vi "exnFormulaBlock Express Formula Template.vi"(0 "X1":waveform(dbl)[](array[waveform]), 1 "X2":waveform(dbl)[](array[waveform]), 2 "X3":waveform(dbl)[](array[waveform]), 3 "X4":waveform(dbl)[](array[waveform]), 5 "X5":waveform(dbl)[](array[waveform]), 7 "X6":waveform(dbl)[](array[waveform]), 9 "X7":waveform(dbl)[](array[waveform]), 11 "error in (no error)":errorcluster, 12 "X8":waveform(dbl)[](array[waveform])) -> (8 "Result":waveform(dbl)[](array[waveform]), 15 "error out":errorcluster)   [LabVIEW 2020]
panel:
  in  "Name Modifier":string="Formula Result"
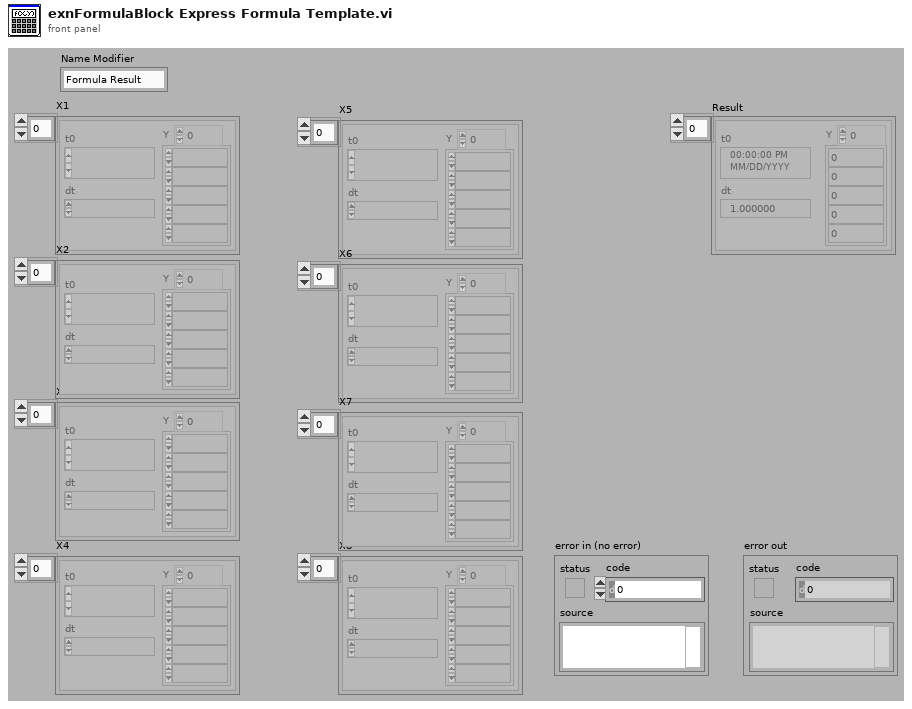
[diagram p1: front panel]
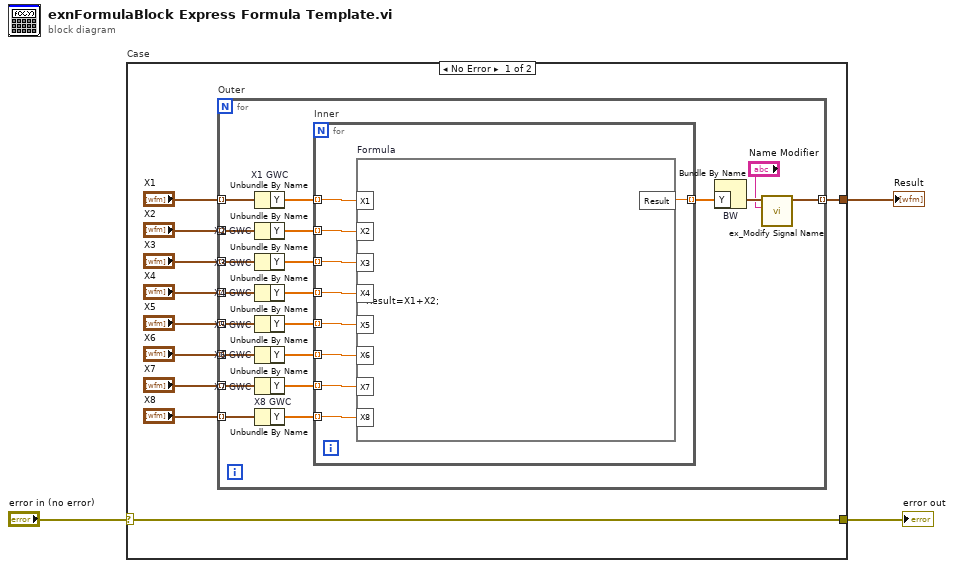
[diagram p0: block diagram]
diagram:
  n1 = case "Case" shown="No Error" "error in (no error)" {
    selector: "error in (no error)" -> [w4 w43]
    tunnel: [w5 _] -> w3
    tunnel: [w4 w43] -> w1
    frame No Error {
      n2 = for "Outer" {
        tunnel: "X1" -> [w33] mode=indexing
        tunnel: "X2" -> [w31] mode=indexing
        tunnel: "X3" -> [w23] mode=indexing
        tunnel: "X4" -> [w22] mode=indexing
        tunnel: "X5" -> [w21] mode=indexing
        tunnel: "X6" -> [w20] mode=indexing
        tunnel: "X7" -> [w19] mode=indexing
        tunnel: "X8" -> [w18] mode=indexing
        tunnel: [w15] -> w5 mode=indexing
        n3 = Unbundle By Name "X1 GWC"(w33) -> ("Y"=w32:dbl[])
        n4 = Unbundle By Name "X2 GWC"(w31) -> ("Y"=w30:dbl[])
        n5 = Unbundle By Name "X3 GWC"(w23) -> ("Y"=w25:dbl[])
        n6 = Unbundle By Name "X4 GWC"(w22) -> ("Y"=w24:dbl[])
        n7 = Unbundle By Name "X5 GWC"(w21) -> ("Y"=w26:dbl[])
        n8 = Unbundle By Name "X6 GWC"(w20) -> ("Y"=w27:dbl[])
        n9 = Unbundle By Name "X7 GWC"(w19) -> ("Y"=w28:dbl[])
        n10 = Unbundle By Name "X8 GWC"(w18) -> ("Y"=w29:dbl[])
        n11 = for "Inner" {
          tunnel: w32 -> [w34] mode=indexing
          tunnel: w30 -> [w42] mode=indexing
          tunnel: w25 -> [w41] mode=indexing
          tunnel: w24 -> [w40] mode=indexing
          tunnel: w26 -> [w39] mode=indexing
          tunnel: w27 -> [w38] mode=indexing
          tunnel: w28 -> [w37] mode=indexing
          tunnel: w29 -> [w36] mode=indexing
          tunnel: [w35] -> w17 mode=indexing
          n12 = formula code="Result=X1+X2;"("X1"=w34, "X2"=w42, "X3"=w41, "X4"=w40, "X5"=w39, "X6"=w38, "X7"=w37, "X8"=w36) -> ("Result"=w35:dbl)
        }
        n13 = Bundle By Name "BW"("Y"=w17) -> (w16:waveform(dbl))  [unwired: 1 in]
        n14 = call <vilib>:"ex_Modify Signal Name.vi"("Name Modifier"="Name Modifier", "waveform in"=w16) -> ("waveform out"=w15:waveform(dbl))  [unwired: 8 in, 1 out]
      }
    }
    frame Error {
    }
  }
  "Result" <- w3
  "error out" <- w1
